vi "hello_world.vi"() -> ()   [LabVIEW 2019]
panel:
  in  "Numeric 2":dbl
  in  "Numeric 1":dbl
  out "Numeric 3":dbl
  out "String Output":string
  in  "String Input":string
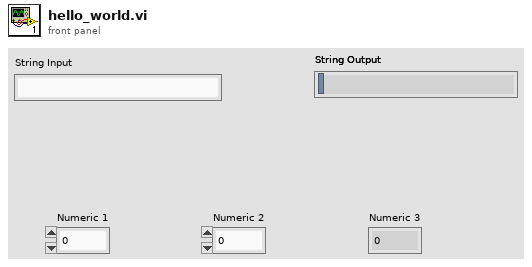
[diagram p1: front panel]
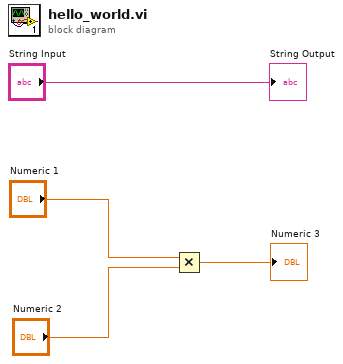
[diagram p0: block diagram]
diagram:
  n1 = Multiply(x="Numeric 1", y="Numeric 2") -> (x*y=→"Numeric 3":dbl)
  "String Output" <- "String Input"
